vi "test Get-Set-Get Label Properties.vi"(8 "error in":errorcluster, 11 "TestCase in":refnum<class "Scripting.lvclass">) -> (0 "error out":errorcluster, 3 "TestCase out":refnum<class "Scripting.lvclass">)   [LabVIEW 2020, in "Scripting.lvclass"]
uses:
  Scripting.lvclass
  <vilib>/addons/_JKI Toolkits/VI Tester/TestCase.llb/TestCase.lvclass
  Scripting/AIM/AIM ARINC 429 Scripting.lvlib
  Shared/Label Properties.ctl
  Shared/Label.ctl
  Shared/Direction.ctl
  Shared/SDI.ctl
  Shared/Transfer Type.ctl
  C:/Program Files (x86)/National Instruments/LabVIEW 2020/vi.lib/addons/_JKI Toolkits/VI Tester/TestCase.llb/TestCase.lvclass
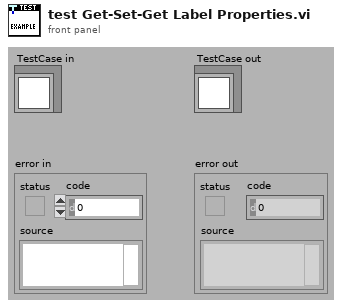
[diagram p1: front panel]
types:
  T1 = typedef "Transfer Type.ctl" = enum16{"Scheduled", "Acyclic", "Block", "Strobe"}
  T2 = typedef "Direction.ctl" = enum16{"Rx", "Tx"}
  T3 = typedef "SDI.ctl" = i32
  T4 = typedef "Label Properties.ctl" = cluster{"label (Dec)":T5, "SDI value":u8, "SDI enabled":bool}
  T5 = typedef "Label.ctl" = u8
  T6 = typedef "Custom Device API.lvlib/Custom Device Item Ref.ctl" = u64
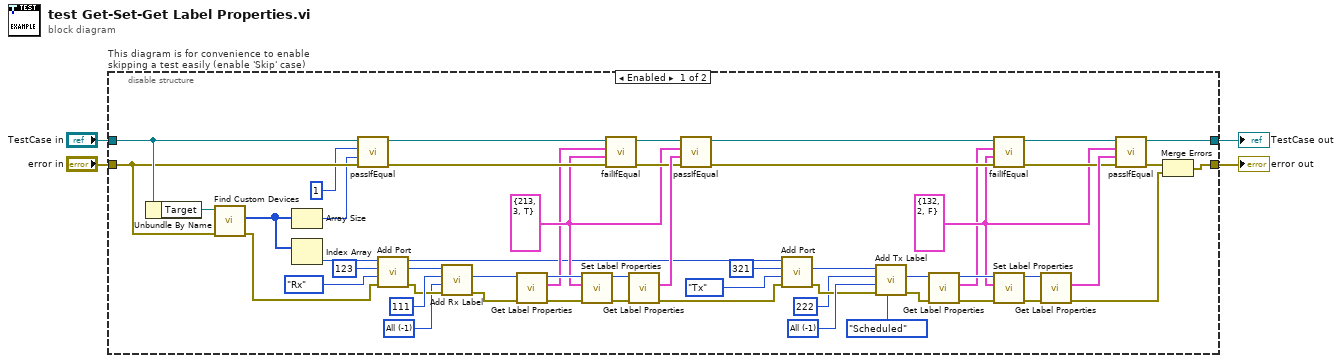
[diagram p0: block diagram]
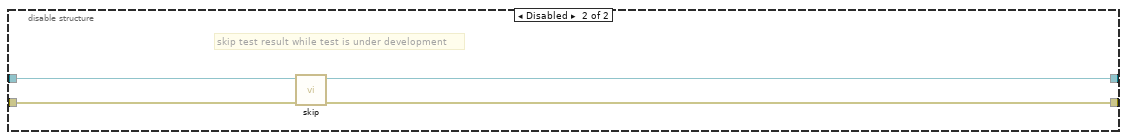
[diagram p2: hidden frame]
diagram:
  n1 = disable-structure "This diagram is for convenience to enable skipping a test easily (enable 'Skip' case)" shown="Enabled" {
    disable-tunnel: "TestCase in" -> [w56 w61]
    disable-tunnel: [w50 w59] -> w1
    disable-tunnel: [w52 w60] -> w3
    disable-tunnel: "error in" -> [w55 w58]
    frame Enabled {
      w15 = T3 -1 items=["All"=-1, "0 (b00)"=0, "1 (b01)"=1, "2 (b10)"=2, "3 (b11)"=3] ("SDI value")
      w18 = T3 -1 items=["All"=-1, "0 (b00)"=0, "1 (b01)"=1, "2 (b10)"=2, "3 (b11)"=3] ("SDI value")
      w28 = T4 {"label (Dec)"=132, "SDI value"=2, "SDI enabled"=FALSE} ("label properties")
      w34 = T4 {"label (Dec)"=213, "SDI value"=3, "SDI enabled"=TRUE} ("label properties")
      n2 = Unbundle By Name(w56) -> ("Target"=w57:refnum<k24>)
      n3 = call "Find Custom Devices.vi"("error in"=w55, "target in"=w57) -> ("error out"=w24:errorcluster, "AIM ARINC 429 custom devices"=w26:u64[])  [unwired: 7 in, 1 out]
      n4 = Array Size(array=w26) -> (size(s)=w53:i32)
      n5 = Index Array(array=w26) -> (element=w25:u64)  [unwired: 1 in]
      n6 = call-dynamic "passIfEqual.vi"("error in (no error)"=w55, "y"=w53, "x"=1 ("size(s)"), "TestCase in"=w56) -> ("error out"=w37:errorcluster, "TestCase out"=w38:refnum<class "Scripting.lvclass">)  [unwired: 6 in]
      n7 = call "Add Port.vi"("error in"=w24, "direction"=Direction."Rx", "port number"=u16 123, "AIM ARINC 429 custom device in"=w25) -> ("error out"=w19:errorcluster, "port"=w21:T6, "AIM ARINC 429 custom device out"=w9:T6)  [unwired: 5 in]
      n8 = call "Add Rx Label.vi"("error in"=w19, "SDI value"=w18, "label value"=u32 111, "port in"=w21) -> ("error out"=w17:errorcluster, "label"=w16:T6)  [unwired: 5 in, 1 out]
      n9 = call "Get Label Properties.vi"("error in"=w17, "label ref in"=w16) -> ("error out"=w48:errorcluster, "label properties"=w33:T4, "label ref out"=w49:T6)  [unwired: 6 in, 1 out]
      n10 = call "Set Label Properties.vi"("error in"=w48, "label properties"=w34, "label ref"=w49) -> ("error out"=w46:errorcluster, "label ref out"=w47:T6)  [unwired: 7 in]
      n11 = call-dynamic "failIfEqual.vi"("error in (no error)"=w37, "y"=w34, "x"=w33, "TestCase in"=w38) -> ("error out"=w35:errorcluster, "TestCase out"=w36:refnum<class "Scripting.lvclass">)  [unwired: 6 in]
      n12 = call "Get Label Properties.vi"("error in"=w46, "label ref in"=w47) -> ("error out"=w8:errorcluster, "label properties"=w45:T4)  [unwired: 6 in, 2 out]
      n13 = call-dynamic "passIfEqual.vi"("error in (no error)"=w35, "y"=w45, "x"=w34, "TestCase in"=w36) -> ("error out"=w31:errorcluster, "TestCase out"=w32:refnum<class "Scripting.lvclass">)  [unwired: 6 in]
      n14 = call "Add Port.vi"("error in"=w8, "direction"=Direction."Tx", "port number"=u16 321, "AIM ARINC 429 custom device in"=w9) -> ("error out"=w14:errorcluster, "port"=w12:T6)  [unwired: 5 in, 1 out]
      n15 = call "Add Tx Label.vi"("transfer type"=Transfer_Type."Scheduled", "error in"=w14, "SDI value"=w15, "label value"=u32 222, "port in"=w12) -> ("error out"=w7:errorcluster, "label"=w6:T6)  [unwired: 4 in, 1 out]
      n16 = call "Get Label Properties.vi"("error in"=w7, "label ref in"=w6) -> ("error out"=w42:errorcluster, "label properties"=w27:T4, "label ref out"=w41:T6)  [unwired: 6 in, 1 out]
      n17 = call-dynamic "failIfEqual.vi"("error in (no error)"=w31, "y"=w28, "x"=w27, "TestCase in"=w32) -> ("error out"=w29:errorcluster, "TestCase out"=w30:refnum<class "Scripting.lvclass">)  [unwired: 6 in]
      n18 = call "Set Label Properties.vi"("error in"=w42, "label properties"=w28, "label ref"=w41) -> ("error out"=w44:errorcluster, "label ref out"=w43:T6)  [unwired: 7 in]
      n19 = call "Get Label Properties.vi"("error in"=w44, "label ref in"=w43) -> ("error out"=w40:errorcluster, "label properties"=w39:T4)  [unwired: 6 in, 2 out]
      n20 = call-dynamic "passIfEqual.vi"("error in (no error)"=w29, "y"=w39, "x"=w28, "TestCase in"=w30) -> ("error out"=w51:errorcluster, "TestCase out"=w50:refnum<class "Scripting.lvclass">)  [unwired: 6 in]
      n21 = Merge Errors(w51, w40) -> (w52:errorcluster)
    }
    frame Disabled {
      # "skip test result while test is under development"
      n22 = call <vilib>:"skip.vi"("error in (no error)"=w58, "TestCase in"=w61) -> ("error out"=w60:errorcluster, "TestCase out"=w59:refnum<class "Scripting.lvclass">)  [unwired: 8 in]
    }
  }
  "error out" <- w3
  "TestCase out" <- w1
